vi "DeQ State.vi"(8 "error in (no error)":errorcluster, 11 "Storage Line in":refnum<class "Storage Line.lvclass">) -> (0 "error out":errorcluster, 1 "timed out?":bool, 2 "State":u16, 3 "Storage Line out":refnum<class "Storage Line.lvclass">)   [LabVIEW 2015, in "cRIO-Carbondioxide.lvlib" / "CO2-Actor.lvlib" / "Storage Line.lvclass"]
uses:
  Storage Line.lvclass
  Storage Line.lvclass/Storage Line.ctl
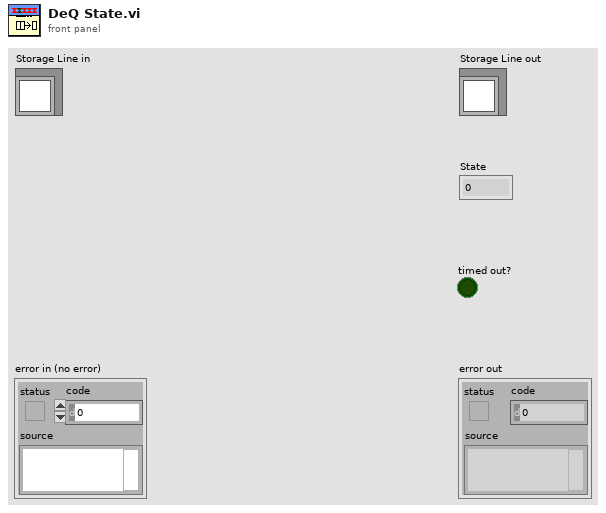
[diagram p1: front panel]
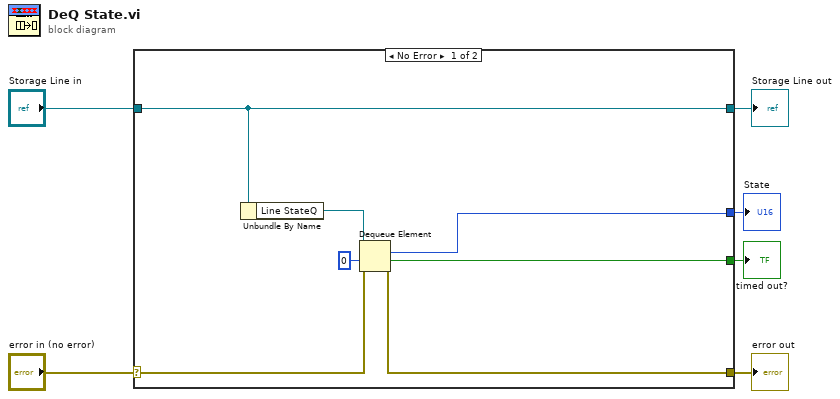
[diagram p0: block diagram]
diagram:
  n1 = case shown="No Error" "error in (no error)" {
    selector: "error in (no error)" -> [w11 w15]
    tunnel: [w10 w15] -> w5
    tunnel: [w13 w14] -> w3
    tunnel: "Storage Line in" -> [w13 w14]
    tunnel: [w8 _] -> w2
    tunnel: [w7 _] -> w1
    frame No Error {
      n2 = Unbundle By Name(w13) -> ("Line StateQ"=w12:refnum<queue>)
      n3 = Dequeue Element(queue=w12, timeout in ms (-1)=0, error in (no error)=w11) -> (element=w7:u16, timed out?=w8:bool, error out=w10:errorcluster)  [unwired: 1 out]
    }
    frame Error {
    }
  }
  "error out" <- w5
  "Storage Line out" <- w3
  "timed out?" <- w2
  "State" <- w1
